vi "Generate Async Msg Event.vi"(7 "AdHoc Msg (\"\")":string, 8 "error in (no error)":errorcluster, 9 "vData":variant, 10 "AsyncMsg":T1, 11 "Main in":refnum<class "Main.lvclass">) -> (0 "error out":errorcluster, 3 "Main out":refnum<class "Main.lvclass">)   [LabVIEW 2019, in "Main.lvclass"]
doc: "Developed by Kevin Thompson\nkevin@thompsonengineering.net\n\nCopyright 2018\nThompson Engineering, LLC"
uses:
  Main.lvclass
  Common/DataTypes/TD Async CmdMsg EventData--cluster.ctl
  DataTypes/AsynMsg_Main--enum.ctl
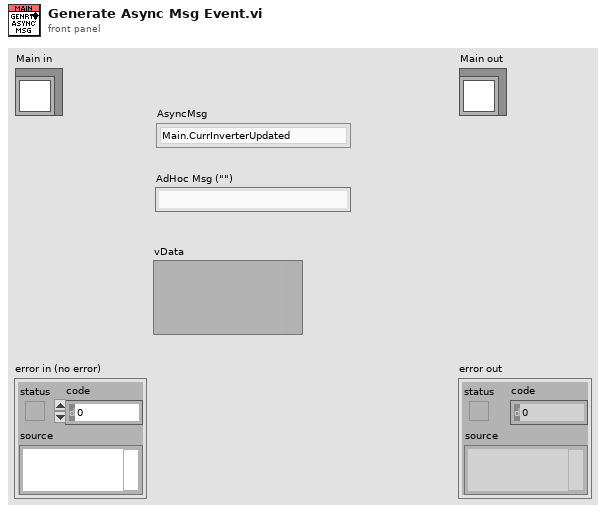
[diagram p1: front panel]
types:
  T1 = typedef "Main.lvclass/AsynMsg_Main--enum.ctl" = enum16{"Main.CurrInverterUpdated"}
  T2 = typedef "TD Async CmdMsg EventData--cluster.ctl" = cluster{"Time Stamp":timestamp, "CmdMsg":string, "vData":variant}
  T3 = typedef "Main.lvclass/Public Events--cluster.ctl" = cluster{"Main.AsyncCmd Event":refnum<user-event>, "Main.AsyncMsg Event":refnum<user-event>, "stop process":refnum<user-event>, "UpdateControlValue Ev":refnum<user-event>, "ProcessingStateChg Ev":refnum<user-event>}
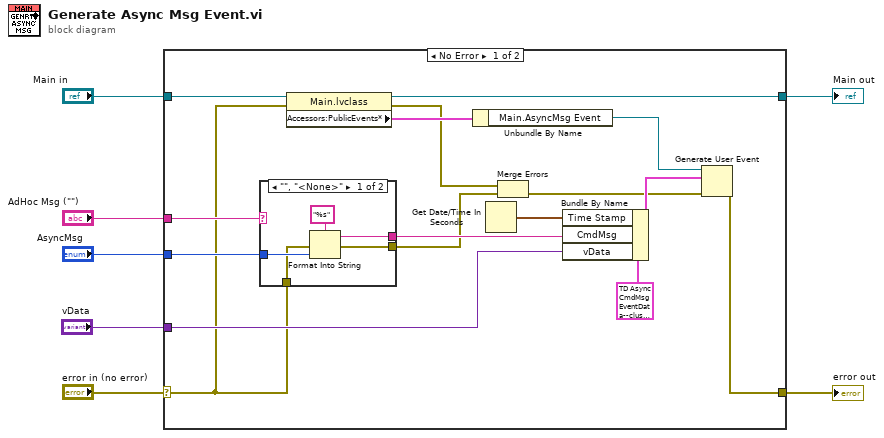
[diagram p0: block diagram]
diagram:
  n1 = case shown="No Error" "error in (no error)" {
    selector: "error in (no error)" -> [w11 w32]
    tunnel: [w23 w32] -> w2
    tunnel: [w12 w31] -> w6
    tunnel: "Main in" -> [w13 w31]
    tunnel: "AsyncMsg" -> [w16 _]
    tunnel: "vData" -> [w18 _]
    tunnel: "AdHoc Msg (\"\")" -> [w15 _]
    frame No Error {
      n2 = case shown="\"\", \"<None>\"" w15 {
        selector: w15 -> [_ w29]
        tunnel: w16 -> [w27 _]
        tunnel: [w26 w29] -> w19
        tunnel: w11 -> [w25 w30]
        tunnel: [w24 w30] -> w17
        frame "", "<None>" {
          n3 = Format Into String(format string="%s", error in=w25, w27) -> (resulting string=w26:string, error out=w24:errorcluster)  [unwired: 1 in]
        }
        frame Default {
        }
      }
      n4 = property class="Main.lvclass"(reference=w13, error in=w11) -> (reference out=w12:refnum<class "Main.lvclass">, error out=w9:errorcluster, "Accessors:PublicEvents*"=w14:T3)
      n5 = Unbundle By Name(w14) -> ("Main.AsyncMsg Event"=w8:refnum<user-event>)
      n6 = Get Date/Time In Seconds() -> (seconds since 1Jan1904=w20:timestamp)
      n7 = Merge Errors(w9, w17) -> (w10:errorcluster)
      n8 = Bundle By Name(cluster=T2 {"Time Stamp"=timestamp(0 s since 1904-01-01), "CmdMsg"="", "vData"=variant} ("Async EvData"), "Time Stamp"=w20, "CmdMsg"=w19, "vData"=w18) -> (w22:T2)
      n9 = Generate User Event(user event=w8, event data cluster=w22, error in=w10) -> (error out=w23:errorcluster)  [unwired: 1 in, 1 out]
    }
    frame Error {
    }
  }
  "error out" <- w2
  "Main out" <- w6
